vi "SetShutterState.vi"(8 "error in (no error)":errorcluster, 10 "Shutter State":T1, 11 "OPA":refnum<class "OPA.lvclass">) -> (0 "error out":errorcluster, 3 "OPA out":refnum<class "OPA.lvclass">)   [LabVIEW 2017, in "OPA.lvclass"]
doc: "---------------------------------------------------------------\nJKI State Machine Objects™\nhttp://jki.net/state-machine-objects/\nCopyright (C) 2005-2015, JKI <info@jki.net>\nALL RIGHTS RESERVEDJKI State Machine Objects (SMO) 1.0.0.4\nJKI - JKI\nCopyright (c) 2015, JKI"
uses:
  OPA.lvclass
  Typedefs/PrivateEvents--OPA.SetShutterState.ctl
  OPA.lvclass/OPA.ctl
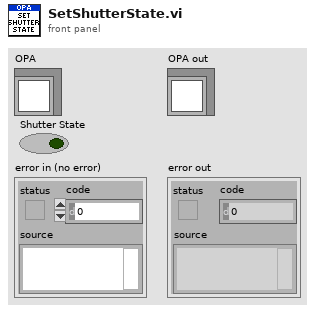
[diagram p1: front panel]
types:
  T1 = typedef "OPA.lvclass/PrivateEvents--OPA.SetShutterState.ctl" = bool
  T2 = typedef "OPA.lvclass/PrivateData--Ref.ctl" = refnum<data-value>
  T3 = typedef "OPA.lvclass/PrivateData--Cluster.ctl" = cluster{"Configuration":T4, "Public Events":T5, "Private Events":T6}
  T4 = typedef "OPA.lvclass/Configuration--Cluster.ctl" = cluster{"Serial Number":string}
  T5 = typedef "OPA.lvclass/PublicEvents--Cluster.ctl" = cluster{"Data Changed":refnum<user-event>}
  T6 = typedef "OPA.lvclass/PrivateEvents--Cluster.ctl" = cluster{"SetWavelength":refnum<user-event>, "SetShutterState":refnum<user-event>}
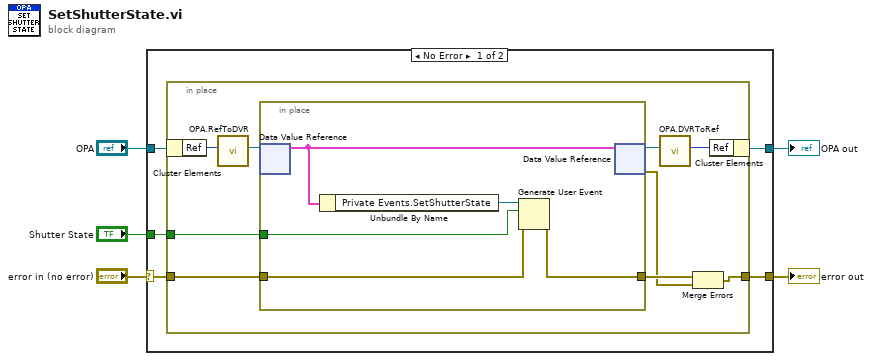
[diagram p0: block diagram]
diagram:
  n1 = case shown="No Error" "error in (no error)" {
    selector: "error in (no error)" -> [w8 w26]
    tunnel: [w7 w26] -> w4
    tunnel: [w9 w25] -> w5
    tunnel: "OPA" -> [w10 w25]
    tunnel: "Shutter State" -> [w6 _]
    frame No Error {
      n2 = in-place {
        in-place-border: w8 -> [w19]
        in-place-border: [w16] -> w7
        in-place-border: w6 -> [w13]
        n3 = in-place-cluster #1(w10) -> ("Ref"=w15:u32)
        n4 = call "OPA.RefToDVR.vi"("Ref"=w15) -> ("Ref"=w12:T2)  [unwired: 10 in]
        n5 = in-place {
          in-place-border: w19 -> [w22]
          in-place-border: [w21] -> w18
          in-place-border: w13 -> [w20]
          n6 = in-place-dvr #2(w12) -> (w24:T3)  [unwired: 1 out]
          n7 = Unbundle By Name(w24) -> ("Private Events.SetShutterState"=w23:refnum<user-event>)
          n8 = Generate User Event(user event=w23, event data cluster=w20, error in=w22) -> (error out=w21:errorcluster)  [unwired: 1 in, 1 out]
          n9 = in-place-dvr #2(w24) -> (w14:T2, w17:errorcluster)
        }
        n10 = call "OPA.DVRToRef.vi"("Ref"=w14) -> ("Ref"=w11:u32)  [unwired: 10 in]
        n11 = Merge Errors(w18, w17) -> (w16:errorcluster)
        n12 = in-place-cluster #1("Ref"=w11) -> (w9:refnum<class "OPA.lvclass">)
      }
    }
    frame Error {
    }
  }
  "error out" <- w4
  "OPA out" <- w5
